vi "Write Snapshot Plot.vi"(8 "error in":errorcluster, 10 "Snapshot Plot":refnum<vi>, 11 "AnalogInput in":refnum<class "AnalogInput.lvclass">) -> (0 "error out":errorcluster, 3 "AnalogInput out":refnum<class "AnalogInput.lvclass">)   [LabVIEW 2019, in "AnalogInput.lvlib" / "AnalogInput.lvclass"]
uses:
  Library/AnalogInput.lvclass
  Library/AnalogInput.lvclass/AnalogInput.ctl
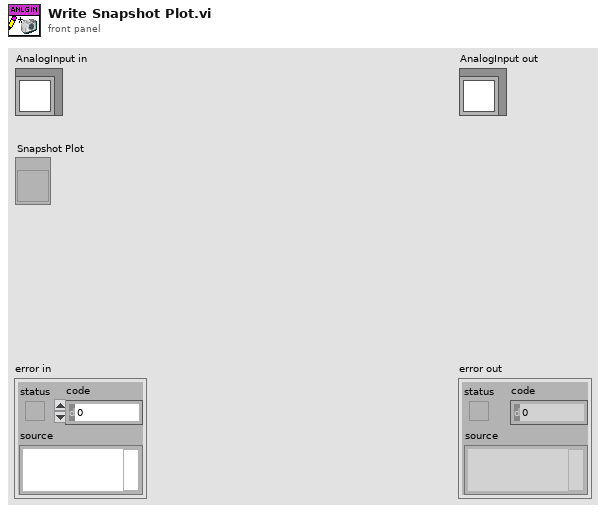
[diagram p1: front panel]
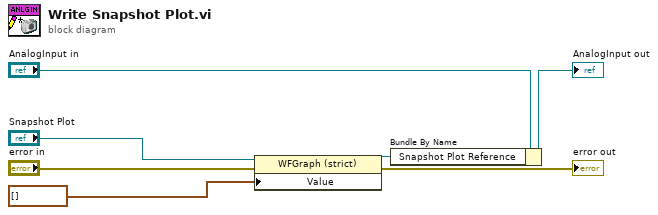
[diagram p0: block diagram]
diagram:
  n1 = property class="WFGraph (strict)"(reference="Snapshot Plot", error in="error in", "Value"=waveform(dbl)[] []) -> (reference out=w4:refnum<vi>, error out=→"error out":errorcluster)
  n2 = Bundle By Name(cluster="AnalogInput in", "Snapshot Plot Reference"=w4) -> (→"AnalogInput out":refnum<class "AnalogInput.lvclass">)
